vi "Thermometer (Demo).vi"(1 "Temp Scale":bool) -> (0 "Temperature":dbl(slide) scale=0.0..100.0 scale format="%.1f")   [LabVIEW 2010]
doc: "This VI simulates measuring a temperature using the temperature sensor on the DAQ Signal Accessory.\n\nIf you have a DAQ board or a DAQ Signal Accessory, then use the Thermometer VI instead."
panel:
  # "deg C\n\ndeg F"
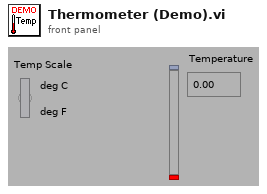
[diagram p1: front panel]
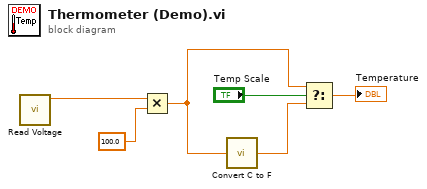
[diagram p0: block diagram]
diagram:
  n1 = call "Read Voltage.vi"() -> ("voltage"=w1:dbl)  [unwired: 6 in, 1 out]
  n2 = Multiply(x=w1, y=100.0) -> (x*y=w2:dbl)
  n3 = call "Convert C to F.vi"("deg C"=w2) -> ("deg F"=w5:dbl)
  n4 = Select(t=w2, s="Temp Scale", f=w5) -> (s? t:f=→"Temperature":dbl)
